vi "SaveCSV.vi"(9 "数据行":string[](array[string]), 10 "表头":string[](array[string]), 11 "Savepath":path) -> (3 "new file path (Not A Path if cancelled)":path)   [LabVIEW 2018]
uses:
  <vilib>/Utility/file.llb/Write Delimited Spreadsheet (string).vi
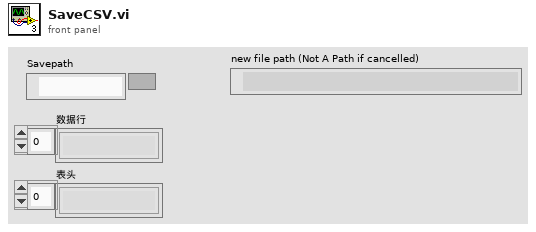
[diagram p1: front panel]
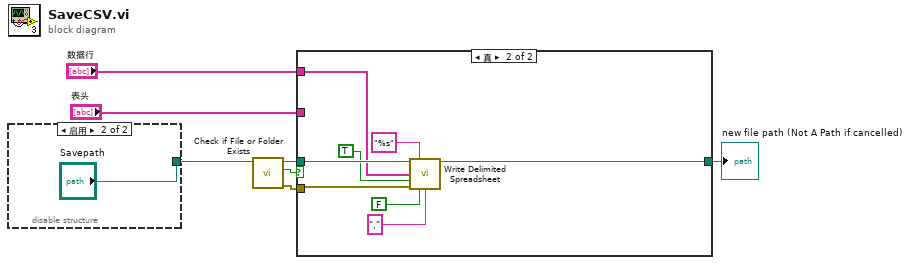
[diagram p0: block diagram]
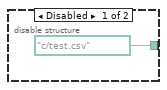
[diagram p2: hidden frame]
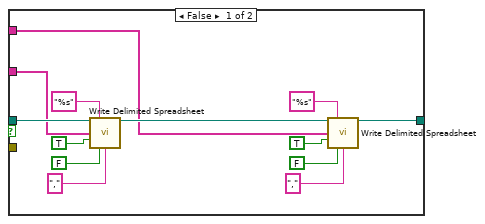
[diagram p3: hidden frame]
diagram:
  n1 = disable-structure shown="启用" {
    disable-tunnel: [path "c:/test.csv" ("path") "Savepath"] -> w7
    frame Disabled {
    }
    frame Enabled {
    }
  }
  n2 = call <vilib>:"Check if File or Folder Exists.vi"("path"=w7) -> ("error out"=w5:errorcluster, "file or folder exists?"=w4:bool, "dup path"=w6:path)  [unwired: 8 in]
  n3 = case shown="真" w4 {
    tunnel: w6 -> [w18 w30]
    tunnel: w5 -> [_ w29]
    tunnel: "表头" -> [w12 _]
    tunnel: [w11 w24] -> w1
    tunnel: "数据行" -> [w10 w23]
    frame False {
      n4 = call-poly <vilib>:"Write Delimited Spreadsheet.vi"("file path (dialog if empty)"=w18, "format (%s)"="%s", "1D data"=w12, "append to file? (new file:F)"=TRUE, "transpose? (no:F)"=FALSE, "delimiter (\\t)"="," ("delimiter (\\t)")) -> ("new file path (Not A Path if cancelled)"=w13:path)  [unwired: 8 in, 1 out]
      n5 = call-poly <vilib>:"Write Delimited Spreadsheet.vi"("file path (dialog if empty)"=w13, "format (%s)"="%s", "1D data"=w10, "append to file? (new file:F)"=TRUE, "transpose? (no:F)"=FALSE, "delimiter (\\t)"="," ("delimiter (\\t)")) -> ("new file path (Not A Path if cancelled)"=w11:path)  [unwired: 8 in, 1 out]
    }
    frame True {
      n6 = call-poly <vilib>:"Write Delimited Spreadsheet.vi"("file path (dialog if empty)"=w30, "format (%s)"="%s", "1D data"=w23, "append to file? (new file:F)"=TRUE, "error in (no error)"=w29, "transpose? (no:F)"=FALSE, "delimiter (\\t)"="," ("delimiter (\\t)")) -> ("new file path (Not A Path if cancelled)"=w24:path)  [unwired: 7 in, 1 out]
    }
  }
  "new file path (Not A Path if cancelled)" <- w1
